vi "main2.vi"() -> ()   [LabVIEW 2023]
uses:
  <extravilib>/ChannelInstances/Tag-path/Read With Abort.vi
  <extravilib>/ChannelInstances/Tag-a[.](wfm(dbl))/Read With Abort.vi
  <extravilib>/ChannelInstances/Tag-c(bool,i32,str)/Read With Abort.vi
  <extravilib>/ChannelInstances/Tag-bool/Read With Abort.vi
  <extravilib>/ChannelInstances/Tag-path/Write With Abort.vi
  <extravilib>/ChannelInstances/Tag-c(bool,i32,str)/Write With Abort.vi
  <extravilib>/ChannelInstances/Tag-bool/Write With Abort.vi
  <extravilib>/ChannelInstances/Tag-a[.](wfm(dbl))/Write With Abort.vi
  <extravilib>/ChannelInstances/Tag-path/Instantiate.vi
  <extravilib>/ChannelInstances/Tag-a[.](wfm(dbl))/Instantiate.vi
  <extravilib>/ChannelInstances/Tag-c(bool,i32,str)/Instantiate.vi
  <extravilib>/ChannelInstances/Tag-bool/Instantiate.vi
  <extravilib>/ChannelInstances/Tag-path/EndpointRead.vi
  <extravilib>/ChannelInstances/Tag-a[.](wfm(dbl))/EndpointRead.vi
  <vilib>/express/express shared/transition.llb/Dynamic To Waveform Array.vi
  <vilib>/express/express signal manip/GetorSetDDTAttributes/Set DDT Attributes/SetT0.vi
  <vilib>/express/express shared/transition.llb/Waveform Array To Dynamic.vi
  <extravilib>/ChannelInstances/Tag-c(bool,i32,str)/EndpointRead.vi
  <extravilib>/ChannelInstances/Tag-bool/EndpointRead.vi
  <extravilib>/ChannelInstances/Tag-path/Endpoint.vi
  <extravilib>/ChannelInstances/Tag-c(bool,i32,str)/Endpoint.vi
  <extravilib>/ChannelInstances/Tag-bool/Endpoint.vi
  <extravilib>/ChannelInstances/Tag-a[.](wfm(dbl))/Endpoint.vi
  <vilib>/Waveform/WDTFileIO.llb/Export Waveforms To Spreadsheet File (1D).vi
  <vilib>/express/express signal manip/GetorSetDDTAttributes/Set DDT Attributes/Set DDT Properties.xnode
  <vilib>/MakerHub/Toolbox/LMH-Toolbox.lvlib
  <extravilib>/ChannelInstances/Tag-bool.lvlib
  <extravilib>/ChannelInstances/Tag-c(bool,i32,str).lvlib
  <extravilib>/ChannelInstances/Tag-path.lvlib
  <extravilib>/ChannelInstances/Tag-a[.](wfm(dbl)).lvlib
panel:
  out "Numeric":i32
  out "File Location":string
  in  "File  Name":string
  in  "Save":bool
  out "Thermistor Unfiltered 2":waveform(dbl)[](graph)
  out "XY Graph":cluster{timestamp[], "Y":dbl[]}[](graph)
  out "Thermistor Filtered":T1(graph)
  out "Thermistor Unfiltered":T2(graph)
  in  "Thermistor":T3
  out "Waveform Chart 3":T4(graph)
  in  "error in (no error)":errorcluster
  out "error out":errorcluster
  out "Waveform Chart 2":waveform(dbl)(graph)
  out "a0 Scalar":dbl
  out "Waveform Chart":dynamicdata(graph)
  in  "stop":bool
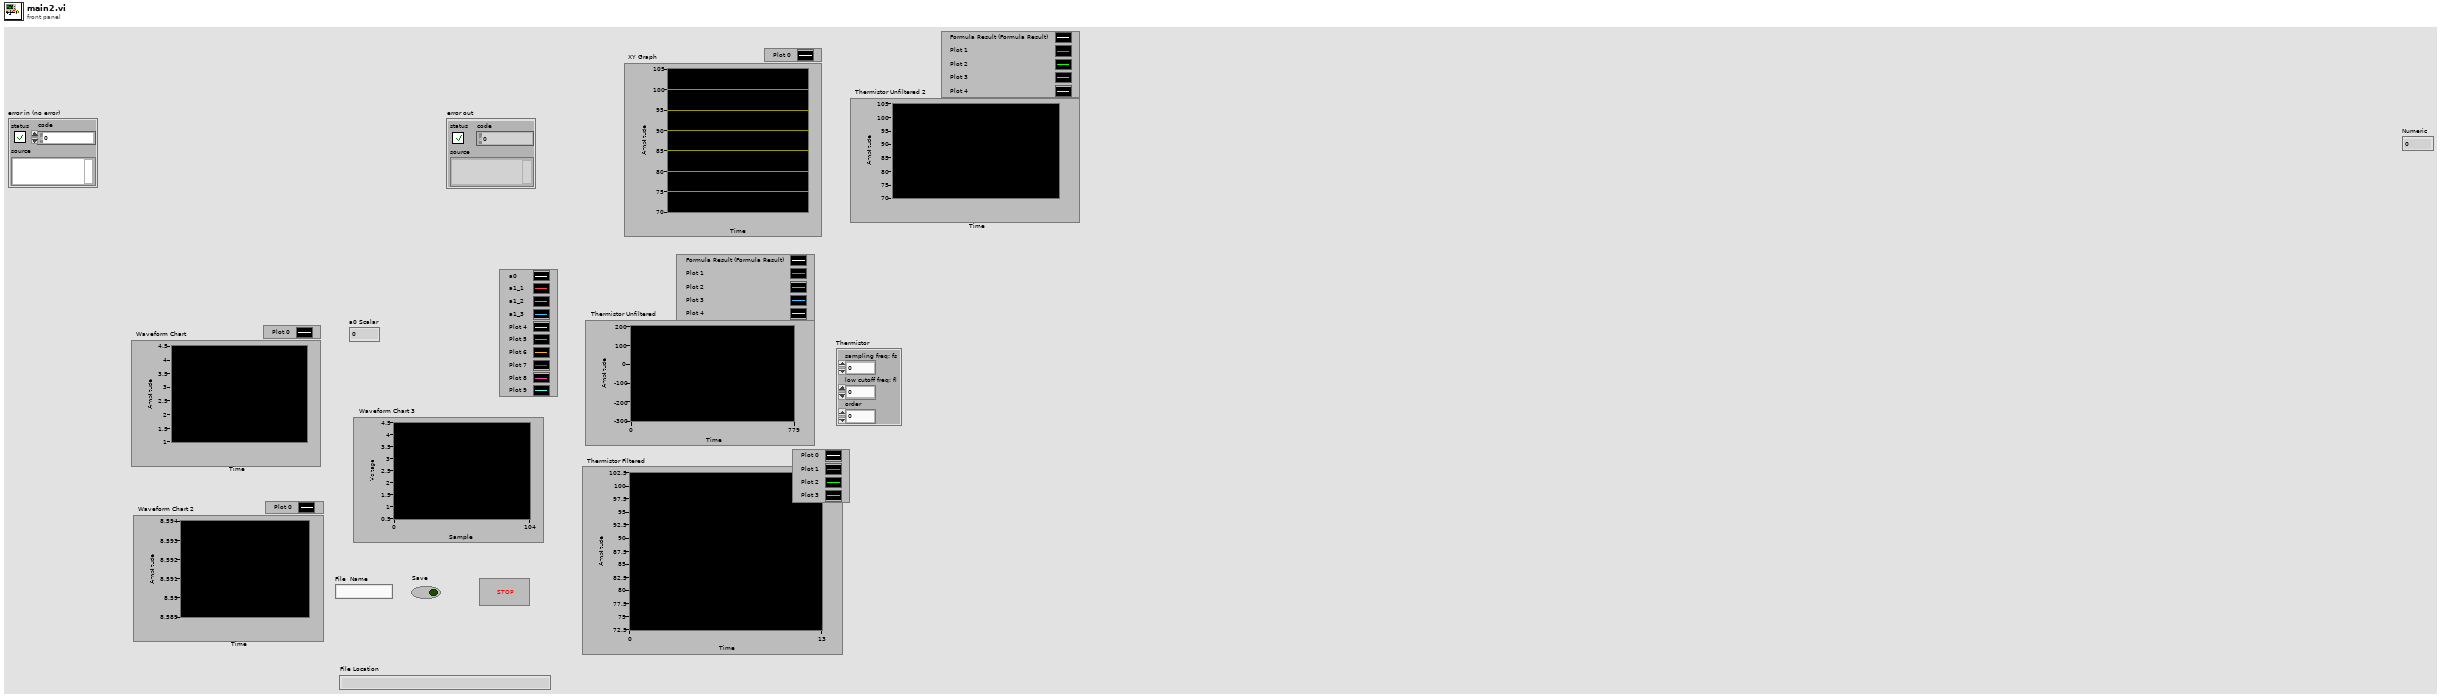
[diagram p1: front panel]
types:
  T1 = cluster{"Temp Filtered[0]":dbl, "Temp Filtered[1]":dbl, "Temp Filtered[2]":dbl, "Temp Filtered[3]":dbl, "Temp Filtered[4]":dbl, "Temp Filtered[5]":dbl, "Temp Filtered[6]":dbl, "Temp Filtered[7]":dbl, "Temp Filtered[8]":dbl}
  T2 = cluster{"[0]":dbl, "[1]":dbl, "[2]":dbl, "[3]":dbl, "[4]":dbl, "[5]":dbl, "[6]":dbl, "[7]":dbl, "[8]":dbl}
  T3 = cluster{"sampling freq: fs":dbl, "low cutoff freq: fl":dbl, "order":i32}
  T4 = cluster{"Data_Array[0]":dbl, "Data_Array[1]":dbl, "Data_Array[2]":dbl, "Data_Array[3]":dbl, "Data_Array[4]":dbl, "Data_Array[5]":dbl, "Data_Array[6]":dbl, "Data_Array[7]":dbl, "Data_Array[8]":dbl}
  T5 = cluster{"Data_Array":dbl[], "Multiplex_Tbl":u32[]}
  T6 = cluster{"Temp[0]":dbl, "Temp[1]":dbl, "Temp[2]":dbl, "Temp[3]":dbl, "Temp[4]":dbl, "Temp[5]":dbl, "Temp[6]":dbl, "Temp[7]":dbl, "Temp[8]":dbl}
  T7 = typedef "Tag-path.lvlib/))Channel.ctl" = refnum<queue>
  T8 = typedef "Tag-a[.](wfm(dbl)).lvlib/))Channel.ctl" = refnum<queue>
  T9 = typedef "Tag-bool.lvlib/))Channel.ctl" = refnum<queue>
  T10 = typedef "Tag-c(bool,i32,str).lvlib/))Channel.ctl" = refnum<queue>
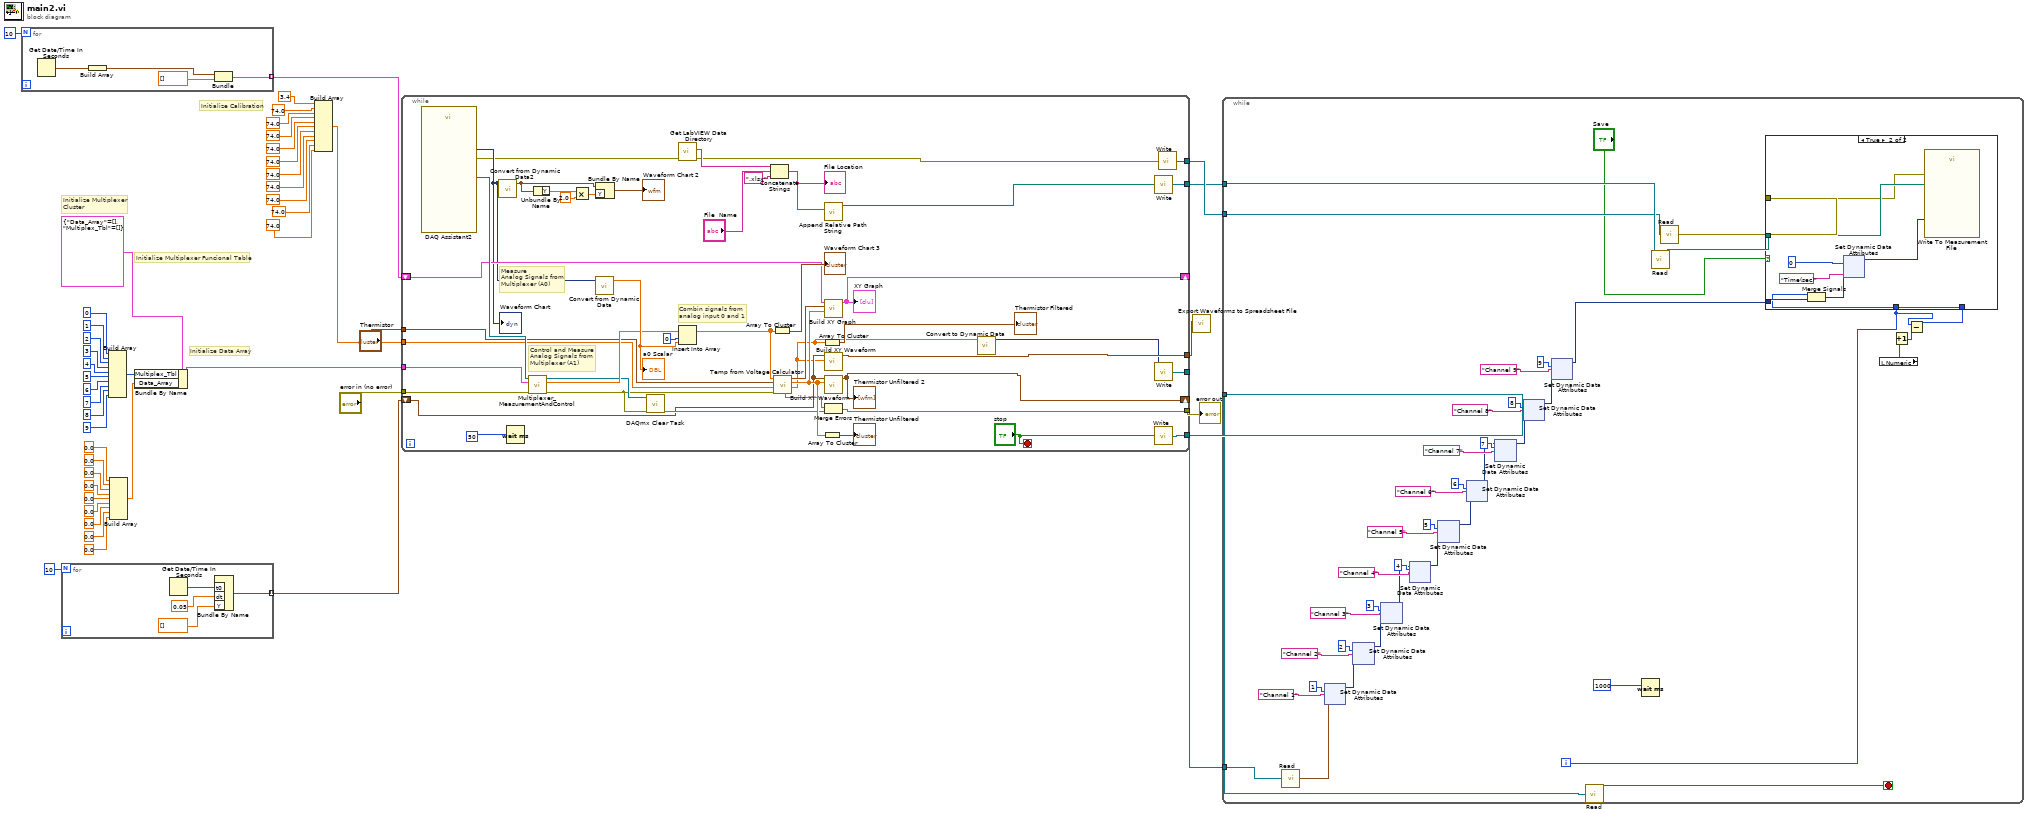
[diagram p0: block diagram]
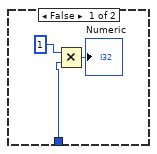
[diagram p2: hidden frame]
diagram:
  # "Initialize Calibration"
  # "Initialize Multiplexer \nCluster"
  # "Initialize Data Array"
  # "Initialize Multiplexer Funcional Table"
  n1 = for {
    N: 10 -> [_]
    tunnel: [w49] -> w35 mode=indexing
    n2 = Get Date/Time In Seconds() -> (seconds since 1Jan1904=w51:timestamp)
    n3 = Build Array(w51) -> (w50:timestamp[])
    n4 = Bundle(w50, "Y"=dbl[] []) -> (w49:cluster{timestamp[], "Y":dbl[]})  [unwired: 1 in]
  }
  n5 = for {
    N: 10 -> [_]
    tunnel: [w52] -> w32 mode=indexing
    n6 = Get Date/Time In Seconds() -> (seconds since 1Jan1904=w54:timestamp)
    n7 = Bundle By Name("t0"=w54, "dt"=0.05, "Y"=dbl[] []) -> (w52:waveform(dbl))  [unwired: 1 in]
  }
  n8 = Build Array(u32 0 ("Waveform"), 1 ("Waveform"), u32 2 ("Waveform"), 3, 4, 5, 6, 7, 8, 9) -> (w37:u32[])
  n9 = Build Array(0.0 ("element"), 0.0 ("element"), 0.0 ("element"), 0.0, 0.0, 0.0, 0.0, 0.0, 0.0) -> (w43:dbl[])
  n10 = Bundle By Name(cluster=T5 {"Data_Array"=[], "Multiplex_Tbl"=[]}, "Multiplex_Tbl"=w37, "Data_Array"=w43) -> (w42:T5)
  n11 = Build Array(3.4 ("element"), 74.0 ("element"), 74.0 ("element"), 74.0 ("element"), 74.0, 74.0, 74.0, 74.0, 74.0, 74.0, 74.0) -> (w27:dbl[])
  n12 = while {
    tunnel: w42 -> [w94]
    tunnel: "error in (no error)" -> [w93]
    tunnel: "Thermistor" -> [w86]
    shift-right: [w82] -> _
    shift-left: w35 -> [w83]
    shift-right: [w58] -> _
    shift-left: w32 -> [w76]
    tunnel: [w60] -> w3
    tunnel: w27 -> [w77]
    tunnel: [w75] -> w26
    tunnel: [w65] -> w5
    tunnel: [w64] -> w4
    tunnel: [w63] -> w1
    tunnel: [w62] -> w2
    stop <- "stop" stop-if-true
    # "Combin signals from \nanalog input 0 and 1"
    # "Measure\nAnalog Signals from\nMultiplexer (A0)"
    # "Control and Measure\nAnalog Signals from\nMultiplexer (A1)"
    n13 = call "DAQ Assistant2"() -> ("task out"=w92:refnum<k21>, "data"=w74:dynamicdata, "error out"=w72:errorcluster)  [unwired: 16 in, 1 out]
    "Waveform Chart" <- w74
    n14 = call "Convert from Dynamic Data2"("Dynamic Data Type"=w74) -> ("Waveform"=w97:waveform(dbl))  [unwired: 3 in]
    n15 = Wait (ms)(milliseconds to wait=50) -> ()  [unwired: 1 out]
    n16 = call "Multiplexer_MeasurementAndControl.vi"("error in (no error)"=w93, "Multiplexer_Cluser"=w94, "Task in"=w92) -> ("error out"=w80:errorcluster, "Data_Array"=w89:dbl[], "Task out"=w87:refnum<k21>)  [unwired: 6 in]
    n17 = Unbundle By Name(w97) -> ("Y"=w99:dbl[])
    n18 = Multiply(x=w99, y=2.0) -> (x*y=w96:dbl[])
    n19 = Bundle By Name(cluster=w97, "Y"=w96) -> (→"Waveform Chart 2":waveform(dbl))
    n20 = call "Convert from Dynamic Data"("Dynamic Data Type"=w74) -> ("Scalar"=w91:dbl)  [unwired: 3 in]
    "a0 Scalar" <- w91
    n21 = call <vilib>:"DAQmx Clear Task.vi"("task in"=w87, "error in"=w80) -> ("error out"=w79:errorcluster)  [unwired: 13 in]
    n22 = call <vilib>:"Get LabVIEW Data Directory.vi"("Error In"=w72) -> ("Error Out"=w66:errorcluster, "LabVIEW Data Path"=w71:string)  [unwired: 9 in]
    n23 = Insert Into Array(array=w89, index=0, new element=w91) -> (w85:dbl[])
    n24 = Concatenate Strings(w71, "File  Name", ".xlsx") -> (w68:string)
    "File Location" <- w68
    n25 = Array To Cluster(array=w85) -> (cluster=→"Waveform Chart 3":T4)
    n26 = call "Temp from Voltage Calculator.vi"("error in (no error)"=w80, "Calibrations"=w77, "Thermistor"=w86, "Data_Array"=w85) -> ("Temp Filtered"=w57:dbl[], "Temp"=w81:dbl[], "Time Read"=w78:timestamp[], "error out"=w73:errorcluster[])  [unwired: 4 in]
    n27 = Array To Cluster(array=w57) -> (cluster=→"Thermistor Filtered":T1)
    n28 = Array To Cluster(array=w81) -> (cluster=→"Thermistor Unfiltered":T6)
    n29 = call <vilib>:"Append Relative Path String.vi"("Relative Path"=w68) -> ("Absolute Path"=w67:path)  [unwired: 9 in, 1 out]
    n30 = call "Build XY Graph.vi"("Meas Temp"=w81, "Meas Time"=w78, "XY In"=w83) -> ("XY out"=w82:cluster{timestamp[], "Y":dbl[]}[])  [unwired: 8 in]
    "XY Graph" <- w82
    n31 = call "Build XY Waveform.vi"("New Temps"=w57, "Waveforms in"=w76) -> ("Waveforms out"=w60:waveform(dbl)[])  [unwired: 9 in]
    n32 = call "Build XY Waveform.vi"("New Temps"=w81, "Waveforms in"=w76) -> ("Waveforms out"=w58:waveform(dbl)[])  [unwired: 9 in]
    "Thermistor Unfiltered 2" <- w58
    n33 = Merge Errors(w73, w79) -> (w75:errorcluster)
    n34 = call "Convert to Dynamic Data"("Array"=w57) -> ("Dynamic Data Type"=w56:dynamicdata)  [unwired: 3 in]
    n35 = call <extravilib>:"Write.vi"("element"=w67) -> ("channel"=w63:T7)  [unwired: 1 out]
    n36 = call <extravilib>:"Write.vi"("element"=w56) -> ("channel"=w62:T8)  [unwired: 1 out]
    n37 = call <extravilib>:"Write.vi"("element"="stop") -> ("channel"=w65:T9)  [unwired: 1 out]
    n38 = call <extravilib>:"Write.vi"("element"=w66) -> ("channel"=w64:T10)  [unwired: 1 out]
  }
  "error out" <- w26
  n39 = call-poly <vilib>:"Export Waveforms to Spreadsheet File.vi"("waveforms"=w3) -> ()  [unwired: 9 in, 2 out]
  n40 = while {
    tunnel: w5 -> [w141]
    tunnel: w4 -> [w112]
    tunnel: w2 -> [w114]
    tunnel: w1 -> [w113]
    i -> [w111]
    stop <- w140 stop-if-true
    n41 = call <extravilib>:"Read.vi"("channel"=w114) -> ("element"=w109:waveform(dbl)[])  [unwired: 1 in, 1 out]
    n42 = xnode "Set Dynamic Data Attributes"("Signals In"=w109, "Signal Index"=1, "Signal Name"="Channel 1") -> ("Signals Out"=w108:dynamicdata)  [unwired: 1 in, 1 out]
    n43 = xnode "Set Dynamic Data Attributes"("Signals In"=w108, "Signal Index"=2, "Signal Name"="Channel 2") -> ("Signals Out"=w107:dynamicdata)  [unwired: 1 in, 1 out]
    n44 = xnode "Set Dynamic Data Attributes"("Signals In"=w107, "Signal Index"=3, "Signal Name"="Channel 3") -> ("Signals Out"=w106:dynamicdata)  [unwired: 1 in, 1 out]
    n45 = xnode "Set Dynamic Data Attributes"("Signals In"=w106, "Signal Index"=4, "Signal Name"="Channel 4") -> ("Signals Out"=w105:dynamicdata)  [unwired: 1 in, 1 out]
    n46 = xnode "Set Dynamic Data Attributes"("Signals In"=w105, "Signal Index"=5, "Signal Name"="Channel 5") -> ("Signals Out"=w104:dynamicdata)  [unwired: 1 in, 1 out]
    n47 = xnode "Set Dynamic Data Attributes"("Signals In"=w104, "Signal Index"=6, "Signal Name"="Channel 6") -> ("Signals Out"=w103:dynamicdata)  [unwired: 1 in, 1 out]
    n48 = xnode "Set Dynamic Data Attributes"("Signals In"=w103, "Signal Index"=7, "Signal Name"="Channel 7") -> ("Signals Out"=w102:dynamicdata)  [unwired: 1 in, 1 out]
    n49 = xnode "Set Dynamic Data Attributes"("Signals In"=w102, "Signal Index"=8, "Signal Name"="Channel 8") -> ("Signals Out"=w101:dynamicdata)  [unwired: 1 in, 1 out]
    n50 = xnode "Set Dynamic Data Attributes"("Signals In"=w101, "Signal Index"=9, "Signal Name"="Channel 9") -> ("Signals Out"=w138:dynamicdata)  [unwired: 1 in, 1 out]
    n51 = call <extravilib>:"Read.vi"("channel"=w141) -> ("element"=w140:bool)  [unwired: 1 in, 1 out]
    n52 = Wait (ms)(milliseconds to wait=1000) -> ()  [unwired: 1 out]
    n53 = call <extravilib>:"Read.vi"("channel"=w113) -> ("element"=w134:path)  [unwired: 1 in, 1 out]
    n54 = call <extravilib>:"Read.vi"("channel"=w112) -> ("element"=w133:errorcluster)  [unwired: 1 in, 1 out]
    n55 = local read "Numeric"() -> (w135:i32)
    n56 = Increment(x=w135) -> (x+1=w136:i32)
    n57 = Subtract(x=w111, y=w136) -> (x-y=w137:i32)
    n58 = case shown="True" "Save" {
      tunnel: w134 -> [_ w269]
      tunnel: w133 -> [_ w268]
      tunnel: w138 -> [_ w267]
      tunnel: w111 -> [w261 _]
      tunnel: w137 -> [_ w266]
      frame False {
        n59 = Multiply(x=1, y=w261) -> (x*y=→"Numeric":i32)
      }
      frame True {
        n60 = Merge Signals(w266, w267) -> (w262:dynamicdata)
        n61 = xnode "Set Dynamic Data Attributes"("Signals In"=w262, "Signal Index"=0, "Signal Name"="Time(sec)") -> ("Signals Out"=w263:dynamicdata)  [unwired: 1 in, 1 out]
        n62 = call "Write To Measurement File"("Signals"=w263, "error in (no error)"=w268, "Filename"=w269) -> ()  [unwired: 14 in, 3 out]
      }
    }
  }
